vi "IsWarning.vi"(4 "Error in":errorcluster) -> (1 "Warning?":bool)   [LabVIEW 2017, in "GPError.lvlib"]
doc: "<B>Warning?</B> will be True only if <B>Error in</B> contains a warning.\n\nThis VI supports appended errors, and <B>Warning?</B> will be True if just a single one of those is a warning.\n\nThis VI is inlined.\n\nSteen Schmidt\nGPower\n16/7 2013"
uses:
  GPError.lvlib
  Typedefs/ErrorType.ctl
panel:
  # "Copyright © 2013\nSteen Schmidt, GPower\nSee enclosed license file for terms and conditions"
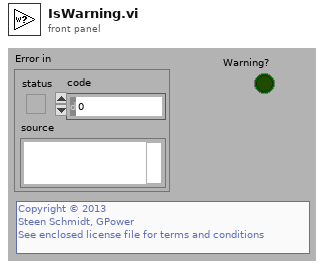
[diagram p1: front panel]
types:
  T1 = typedef "GPError.lvlib/ErrorType.ctl" = enum16{"No Error", "Error", "Warning", "Appended errors", "Appended warnings", "Appended mixed"}
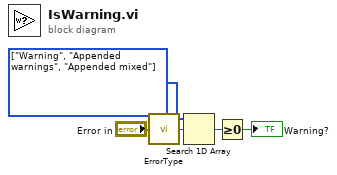
[diagram p0: block diagram]
diagram:
  w2 = T1[] [enum."Warning", enum."Appended warnings", enum."Appended mixed"] items=["No Error", "Error", "Warning", "Appended errors", "Appended warnings", "Appended mixed"]
  n1 = call "ErrorType.vi"("Error in"="Error in") -> ("Error type"=w4:T1)  [unwired: 4 in]
  n2 = Search 1D Array(1D array=w2, element=w4) -> (index of element=w1:i32)  [unwired: 1 in]
  n3 = Greater Or Equal To 0?(x=w1) -> (x >= 0?=→"Warning?":bool)
